vi "arm rate pid.vi"(1 "Rate In":dbl) -> (0 "Rate Out":dbl)   [LabVIEW 2013]
uses:
  <vilib>/addons/control/pid/NI_PID_pid.lvlib
  <vilib>/addons/control/pid/pid.llb/PID Control Input Filter (DBL).vi
  <vilib>/addons/control/pid/pid.llb/PID (DBL).vi
  typedefs/DevRef Type.ctl
  typedefs/fg_typedef.ctl
panel:
  # "A PID to Make the Rate Closed Loop"
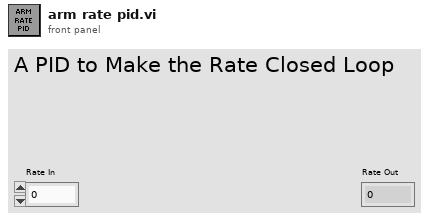
[diagram p1: front panel]
types:
  T1 = typedef "fg_typedef.ctl" = enum16{"Get", "Set"}
  T2 = typedef "DevRef Type.ctl" = enum16{"Shooter Solenoid", "Latch Solenoid", "Right Up Sensor", "Right Down Sensor", "Hold Sensor", "2 Ball Switch", "Arm Encoder"}
  T3 = cluster{"proportional gain (Kc)":dbl, "integral time (Ti, min)":dbl, "derivative time (Td, min)":dbl}
  T4 = typedef "WPI_EncoderDevRef.ctl" = cluster{"DevStatus":errorcluster, "EncoderIndex":T5, "CounterIndex":T6, "DistancePerCount":dbl, "Decoding Type":T7}
  T5 = typedef "FPGA_EncoderIdx.ctl" = enum8{"Enc 0", "Enc 1", "Enc 2", "Enc 3", "Invalid"}
  T6 = typedef "FPGA_CounterCtrSystemIndex.ctl" = enum8{"Ctr 0", "Ctr 1", "Ctr 2", "Ctr 3", "Ctr 4", "Ctr 5", "Ctr 6", "Ctr 7", "Invalid"}
  T7 = typedef "WPI_EncoderType.ctl" = enum16{"1x", "2x", "4x"}
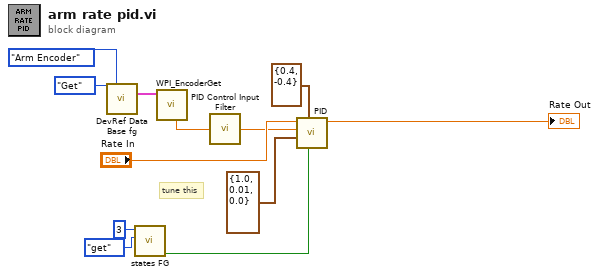
[diagram p0: block diagram]
diagram:
  # "tune this"
  n1 = call "DevRef Data Base fg.vi"(0:fg_typedef."Get" ("Menu"), 10:DevRef_Type."Arm Encoder" ("DevRef to Get")) -> ("Selected Encoder"=w1:T4)  [unwired: 22 in, 3 out]
  n2 = call "states FG.vi"("menu (get)"=enum16{"set", "get"}."get", "Loop ID"=3) -> ("first call?"=w5:bool)  [unwired: 6 in, 3 out]
  n3 = call <vilib>:"WPI_EncoderGet.vi"("EncoderDevRef"=w1) -> ("Rate"=w8:dbl)  [unwired: 5 in, 5 out]
  n4 = call-poly <vilib>:"PID Control Input Filter.vi"("input"=w8) -> ("output"=w10:dbl)  [unwired: 4 in]
  n5 = call-poly <vilib>:"PID.vi"("reinitialize? (F)"=w5, "output range"=cluster{"output high":dbl, "output low":dbl} {"output high"=0.4, "output low"=-0.4}, "PID gains"=T3 {"proportional gain (Kc)"=1.0, "integral time (Ti, min)"=0.01, "derivative time (Td, min)"=0.0}, "process variable"=w10, "setpoint"="Rate In") -> ("output"=→"Rate Out":dbl)  [unwired: 5 in, 1 out]
